vi "Rectangle parameters.vi"(2 "Corners":cluster{"X":sgl, "Y":sgl}[](array[cluster])) -> (16 "Overlay Rectangle Corners":cluster{sgl, sgl, sgl, sgl})   [LabVIEW 2014]
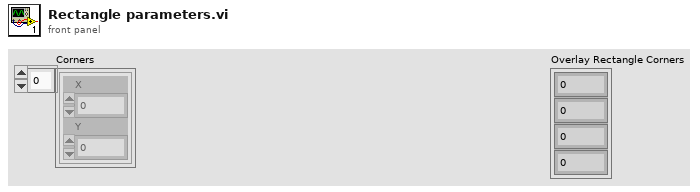
[diagram p1: front panel]
types:
  T1 = cluster{"Corners[0]":cluster{"X":sgl, "Y":sgl}, "Corners[1]":cluster{"X":sgl, "Y":sgl}, "Corners[2]":cluster{"X":sgl, "Y":sgl}, "Corners[3]":cluster{"X":sgl, "Y":sgl}, "Corners[4]":cluster{"X":sgl, "Y":sgl}, "Corners[5]":cluster{"X":sgl, "Y":sgl}, "Corners[6]":cluster{"X":sgl, "Y":sgl}, "Corners[7]":cluster{"X":sgl, "Y":sgl}, "Corners[8]":cluster{"X":sgl, "Y":sgl}}
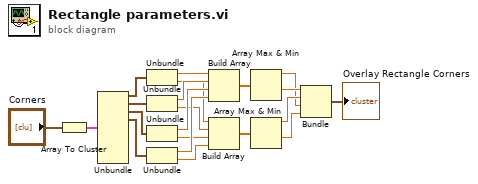
[diagram p0: block diagram]
diagram:
  n1 = Array To Cluster(array="Corners") -> (cluster=w21:T1)
  n2 = Unbundle(w21) -> ("Corners[0]"=w20:cluster{"X":sgl, "Y":sgl}, "Corners[1]"=w19:cluster{"X":sgl, "Y":sgl}, "Corners[2]"=w17:cluster{"X":sgl, "Y":sgl}, "Corners[3]"=w16:cluster{"X":sgl, "Y":sgl})  [unwired: 5 out]
  n3 = Unbundle(w20) -> ("X"=w15:sgl, "Y"=w11:sgl)
  n4 = Unbundle(w19) -> ("X"=w14:sgl, "Y"=w10:sgl)
  n5 = Unbundle(w17) -> ("X"=w13:sgl, "Y"=w9:sgl)
  n6 = Unbundle(w16) -> ("X"=w12:sgl, "Y"=w8:sgl)
  n7 = Build Array(w15, w14, w13, w12) -> (w7:sgl[])
  n8 = Build Array(w11, w10, w9, w8) -> (w6:sgl[])
  n9 = Array Max & Min(array=w7) -> (max value=w3:sgl, min value=w5:sgl)  [unwired: 2 out]
  n10 = Array Max & Min(array=w6) -> (max value=w4:sgl, min value=w2:sgl)  [unwired: 2 out]
  n11 = Bundle(w5, w4, w3, w2) -> (→"Overlay Rectangle Corners":cluster{sgl, sgl, sgl, sgl})  [unwired: 1 in]
